vi "GenerateValidTagSettings.vi"(6 "Minimum tagging period (pws)":u32, 7 "PulseWidth (ms)":dbl, 9 "Minimum tags per file":u32, 10 "Minimum samples per pulse":dbl, 11 "Minimum samples per pulse 2":dbl) -> (0 "TaggingPeriod (pws)":u32, 3 "lower limit":dbl)   [LabVIEW 2017]
uses:
  <vilib>/Utility/error.llb/DialogType.ctl
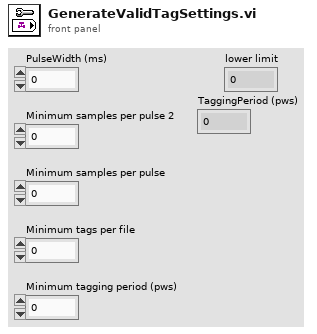
[diagram p1: front panel]
types:
  T1 = typedef "DialogType.ctl" = u16
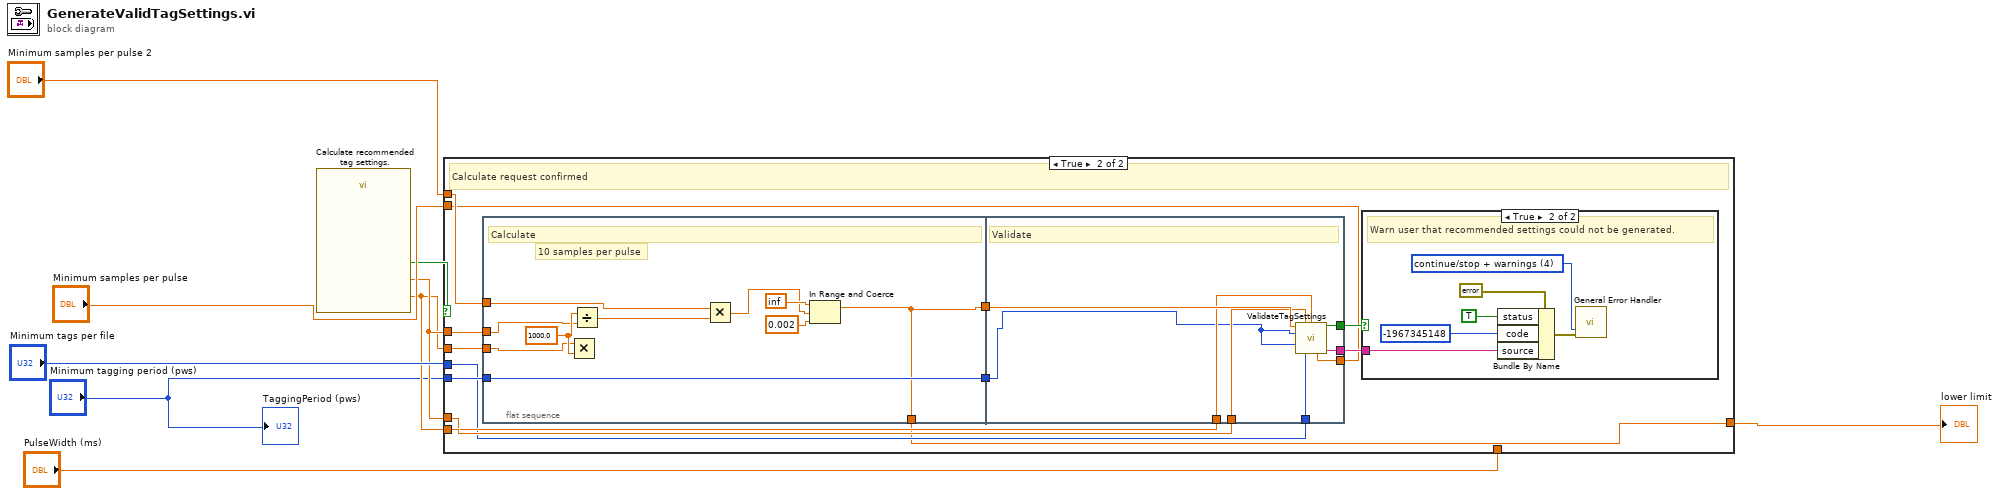
[diagram p0: block diagram]
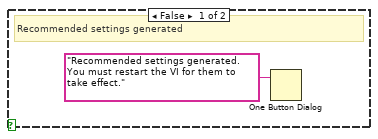
[diagram p3: hidden frame]
diagram:
  n1 = call "Calculate recommended tag settings."() -> ("Minimum file size (s)"=w3:dbl, "Minimum sampling rate (Hz)"=w4:dbl, "Calculate"=w2:bool)  [unwired: 16 in, 1 out]
  n2 = case shown="True" w2 {
    tunnel: w3 -> [_ w23]
    tunnel: w3 -> [_ w20]
    tunnel: w4 -> [_ w19]
    tunnel: w4 -> [_ w17]
    tunnel: "Minimum samples per pulse 2" -> [_ w15]
    tunnel: "Minimum tagging period (pws)" -> [_ w14]
    tunnel: "Minimum tags per file" -> [_ w13]
    tunnel: "Minimum samples per pulse" -> [_ w12]
    tunnel: [w10 w11] -> w8
    tunnel: "PulseWidth (ms)" -> [w10 _]
    frame False {
    }
    frame True {
      # "Calculate request confirmed"
      n3 = flat-sequence {
        tunnel: w23 -> [w28]
        tunnel: w19 -> [w27]
        tunnel: [w24] -> w22
        tunnel: [w25] -> w21
        tunnel: w15 -> [w26]
        tunnel: w14 -> [w25]
        tunnel: [w24] -> w11
        tunnel: w22 -> [w41]
        tunnel: w21 -> [w36]
        tunnel: w20 -> [w40]
        tunnel: [w39] -> w18
        tunnel: w17 -> [w38]
        tunnel: [w37] -> w16
        tunnel: w13 -> [w35]
        tunnel: w12 -> [w34]
        frame #0 {
          w32 = 1000.0
          # "10 samples per pulse"
          # "Calculate"
          n4 = Multiply(x=w28, y=w32) -> ()  [unwired: 1 out]
          n5 = Divide(x=w32, y=w27) -> (x/y=w33:dbl)
          n6 = Multiply(x=w26, y=w33) -> (x*y=w29:dbl)
          n7 = In Range and Coerce(upper limit=inf, x=w29, lower limit=0.002) -> (coerced(x)=w24:dbl)  [unwired: 1 out]
        }
        frame #1 {
          # "Validate"
          n8 = call "ValidateTagSettings.vi"("PulseWidth (ms)"=w41, "Minimum file size (s)"=w40, "Minimum sample rate (Hz)"=w38, "TaggingPeriod (pws)"=w36, "Minimum tagging period (pws)"=w36, "Minimum tags per file"=w35, "Minimum samples per pulse"=w34) -> ("Valid"=w39:bool, "Info"=w37:string)  [unwired: 7 in]
        }
      }
      n9 = case shown="True" w18 {
        tunnel: w16 -> [_ w43]
        frame False {
          # "Recommended settings generated"
          n10 = One Button Dialog(message="Recommended settings generated. You must restart the VI for them to take effect.") -> ()  [unwired: 1 in, 1 out]
        }
        frame True {
          w48 = T1 4 items=["no dialog", "OK message", "continue or stop message", "OK message + warnings", "continue/stop + warnings"] ("type of dialog (OK msg:1)")
          # "Warn user that recommended settings could not be generated."
          n11 = Bundle By Name(cluster=errorcluster {"status"=FALSE, "code"=0, "source"=""} ("error in (no error)"), "status"=TRUE, "code"=-1967345148, "source"=w43) -> (w47:errorcluster)
          n12 = call <vilib>:"General Error Handler.vi"("type of dialog (OK msg:1)"=w48, "error in (no error)"=w47) -> ()  [unwired: 9 in, 5 out]
        }
      }
    }
  }
  "lower limit" <- w8
  "TaggingPeriod (pws)" <- "Minimum tagging period (pws)"
